vi "Get Newest File.vi"(8 "error in (no error)":errorcluster, 11 "files":path[](array[path])) -> (0 "error out":errorcluster, 3 "newest file":path)   [LabVIEW 2018, in "Utilities.lvlib"]
uses:
  Utilities.lvlib
panel:
  # "Connector Pane"
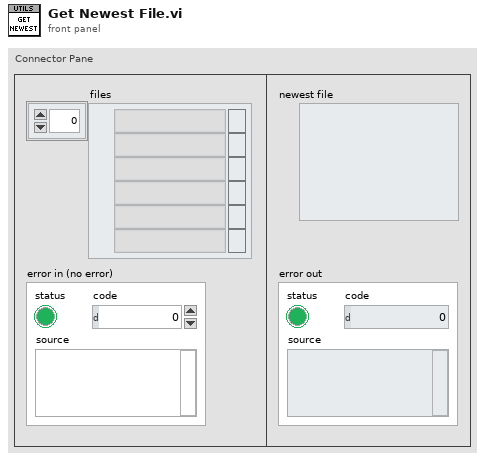
[diagram p1: front panel]
types:
  T1 = cluster{"CreationTimeUtc":timestamp, "File Path":path}
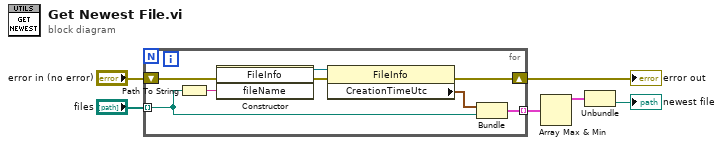
[diagram p0: block diagram]
diagram:
  n1 = for {
    tunnel: "files" -> [w7] mode=indexing
    tunnel: [w11] -> w2 mode=indexing
    shift-right: [w9] -> w6
    shift-left: "error in (no error)" -> [w10]
    n2 = Path To String(path=w7) -> (string=w14:string)
    n3 = constructor class="FileInfo"(error in=w10, "fileName"=w14) -> (reference out=w13:refnum<k24>, error out=w12:errorcluster)  [unwired: 2 in, 2 out]
    n4 = property class="FileInfo"(reference=w13, error in=w12) -> (error out=w9:errorcluster, "CreationTimeUtc"=w8:timestamp)  [unwired: 1 out]
    n5 = Bundle("CreationTimeUtc"=w8, "File Path"=w7) -> (w11:T1)  [unwired: 1 in]
  }
  "error out" <- w6
  n6 = Array Max & Min(array=w2) -> (max value=w3:T1)  [unwired: 3 out]
  n7 = Unbundle(w3) -> ("File Path"=→"newest file":path)  [unwired: 1 out]
